vi "Day 8 Puzzle 2.vi"(11 "Path":path) -> ()   [LabVIEW 2021]
uses:
  <vilib>/Utility/file.llb/Read Delimited Spreadsheet (string).vi
panel:
  out "max value":i32
  out "Scenic Scores":i32[][](array[numeric])
  out "sum":i32
  out "Array":bool[][](array[boolean])
  out "Numeric":i32
  out "Array":bool[][](array[boolean])
  out "Number of rows":i32
  out "Number of columns":i32
  out "Grid array":i32[][](array[numeric])
  out "subarray":string[](array[string])
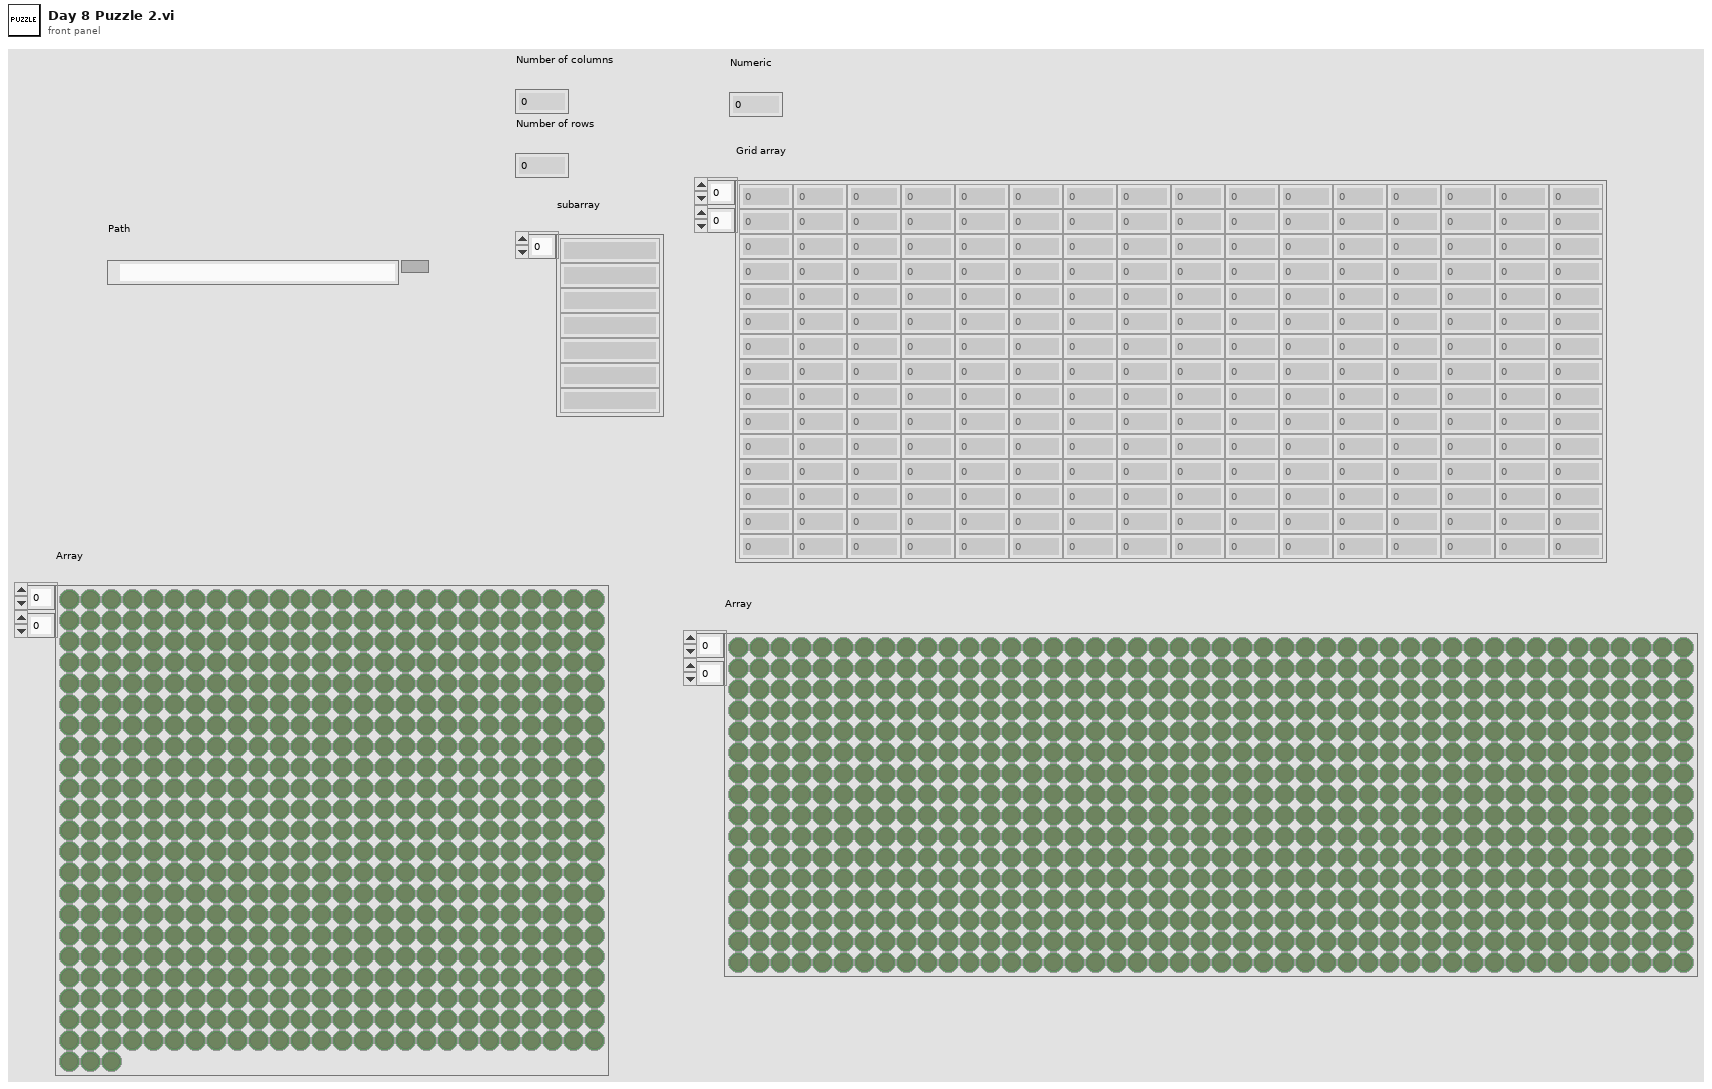
[diagram p1: front panel]
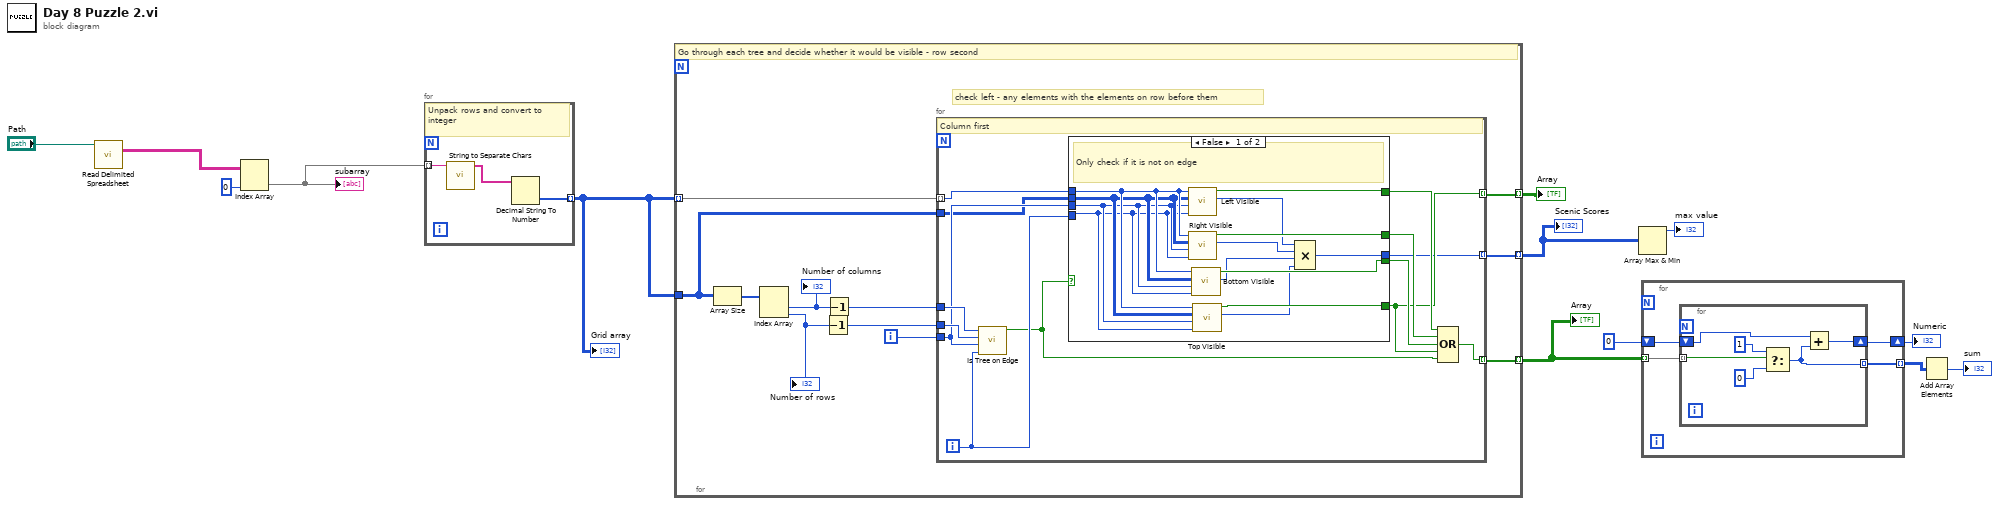
[diagram p0: block diagram]
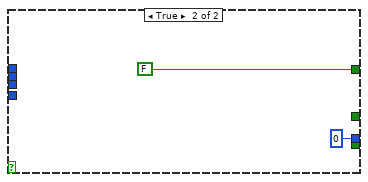
[diagram p2: hidden frame]
diagram:
  n1 = call-poly <vilib>:"Read Delimited Spreadsheet.vi"("file path (dialog if empty)"="Path") -> ("all rows"=w12:string[][])  [unwired: 9 in, 5 out]
  n2 = Index Array(array=w12, index (col)=0 ("disabled index (col)")) -> (element=w10:string[])  [unwired: 1 in]
  "subarray" <- w10
  n3 = for {
    tunnel: w10 -> [w16] mode=indexing
    tunnel: [w14] -> w9 mode=indexing
    # "Unpack rows and convert to integer"
    n4 = call "String to Separate Chars.vi"("String"=w16) -> ("Array"=w15:string[])  [unwired: 10 in]
    n5 = Decimal String To Number(string=w15) -> (number=w14:i32[])  [unwired: 2 in, 1 out]
  }
  "Grid array" <- w9
  n6 = for {
    tunnel: w9 -> [w26] mode=indexing
    tunnel: w9 -> [w19]
    tunnel: [w23] -> w5 mode=indexing
    tunnel: [w18] -> w6 mode=indexing
    tunnel: [w17] -> w2 mode=indexing
    i -> [w22]
    # "check left - any elements with the elements on row before them"
    # "Go through each tree and decide whether it would be visible - row second"
    n7 = Array Size(array=w19) -> (size(s)=w27:i32[])
    n8 = Index Array(array=w27) -> (element #1=w25:i32, element #2=w21:i32)  [unwired: 2 in]
    "Number of columns" <- w25
    "Number of rows" <- w21
    n9 = Decrement(x=w21) -> (x-1=w20:i32)
    n10 = Decrement(x=w25) -> (x-1=w24:i32)
    n11 = for {
      tunnel: w26 -> [w37] mode=indexing
      tunnel: w24 -> [w40]
      tunnel: [w35] -> w23 mode=indexing
      tunnel: w22 -> [w38]
      tunnel: w20 -> [w39]
      tunnel: w19 -> [w36]
      tunnel: [w29] -> w18 mode=indexing
      tunnel: [w28] -> w17 mode=indexing
      i -> [w34]
      # "Column first"
      n12 = call "Is Tree on Edge"("current row"=w34, "corrent column"=w38, "number of rows"=w39, "number of columns"=w40) -> ("Is on edge?"=w33:bool)  [unwired: 7 in]
      n13 = case shown="False" w33 {
        tunnel: w38 -> [w48 _]
        tunnel: w37 -> [w50 _]
        tunnel: w36 -> [w49 _]
        tunnel: [w53 FALSE ("Visible")] -> w31
        tunnel: w34 -> [w47 _]
        tunnel: [w52 _] -> w32
        tunnel: [w51 _] -> w30
        tunnel: [w46 _] -> w29
        tunnel: [w41 0] -> w28
        frame False {
          # "Only check if it is not on edge"
          n14 = call "Left Visible.vi"("Current column"=w47, "Current row"=w48, "Full array"=w49, "Element"=w50) -> ("Viewing Distance"=w45:i32, "Visible"=w53:bool)  [unwired: 6 in]
          n15 = call "Right Visible.vi"("Current column"=w47, "Current row"=w48, "Full array"=w49, "Element"=w50) -> ("Viewing Distance"=w44:i32, "Visible"=w52:bool)  [unwired: 6 in]
          n16 = call "Bottom Visible.vi"("Current column"=w47, "Current row"=w48, "Full array"=w49, "Element"=w50) -> ("Viewing Distance"=w43:i32, "Visible"=w51:bool)  [unwired: 6 in]
          n17 = call "Top Visible.vi"("Current column"=w47, "Current row"=w48, "Full array"=w49, "Element"=w50) -> ("Viewing Distance"=w42:i32, "Visible"=w46:bool)  [unwired: 6 in]
          n18 = Compound Arithmetic op=MULTIPLY(w45, w44, w43, w42) -> (w41:i32)
        }
        frame True {
        }
      }
      n19 = Compound Arithmetic op=OR(w31, w32, w30, w29, w33) -> (w35:bool)
    }
  }
  "Array" <- w5
  "Array" <- w6
  "Scenic Scores" <- w2
  n20 = Array Max & Min(array=w2) -> (max value=→"max value":i32)  [unwired: 3 out]
  n21 = for {
    tunnel: w5 -> [w59] mode=indexing
    shift-right: [w57] -> w7
    shift-left: 0 -> [w58]
    tunnel: [w56] -> w4 mode=indexing
    n22 = for {
      tunnel: w59 -> [w63] mode=indexing
      shift-right: [w61] -> w57
      shift-left: w58 -> [w62]
      tunnel: [w60] -> w56 mode=indexing
      n23 = Select(t=1, s=w63, f=0) -> (s? t:f=w60:i32)
      n24 = Add(x=w62, y=w60) -> (x+y=w61:i32)
    }
  }
  "Numeric" <- w7
  n25 = Add Array Elements(numeric array=w4) -> (sum=→"sum":i32)
